vi "Protocol.Address Lookup Table Initialize.vi"(8 "error in (no error)":errorcluster) -> (0 "error out":errorcluster {"code" min=0 max=0}, 3 "Address LUT":T1)   [LabVIEW 2019, in "J1939 Addon Engine.lvlib"]
uses:
  J1939 Addon Engine.lvlib
  Types/Protocol.Address Table Reference.ctl
  Types/Protocol.Address Lookup Table Action.ctl
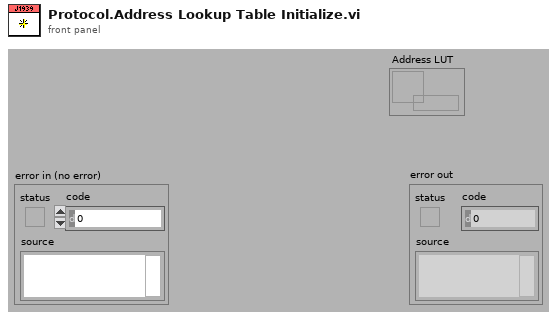
[diagram p1: front panel]
types:
  T1 = typedef "J1939 Addon Engine.lvlib/Protocol.Address Table Reference.ctl" = refnum<data-value>
  T2 = typedef "J1939 Addon Engine.lvlib/Protocol.Address Lookup Table Action.ctl" = enum16{"Initialize", "Add", "Get", "Remove", "Get All"}
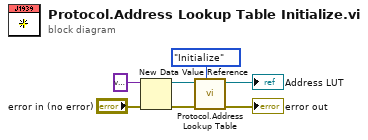
[diagram p0: block diagram]
diagram:
  n1 = New Data Value Reference(data value=variant ("variant"), error in="error in (no error)") -> (data value reference=w5:refnum<data-value>, error out=w4:errorcluster)
  n2 = call "Protocol.Address Lookup Table.vi"("Action"=Protocol.Address_Lookup_Table_Action."Initialize", "error in (no error)"=w4, "Address LUT"=w5) -> ("error out"=→"error out":errorcluster, "Address LUT out"=→"Address LUT":T1)  [unwired: 4 in, 3 out]
